vi "Calc Gain and Offset.vi"(9 "output cluster":T2, 10 "Count":u8, 11 "CalStatus":T1(ring)) -> (2 "New Count":u8, 3 "NewCalStatus":T1(ring))   [LabVIEW 2016]
uses:
  Controls/Cal Refs.ctl
  <vilib>/Analysis/baseanly.llb/Mean (DBL).vi
  <vilib>/Analysis/NI_AALBase.lvlib
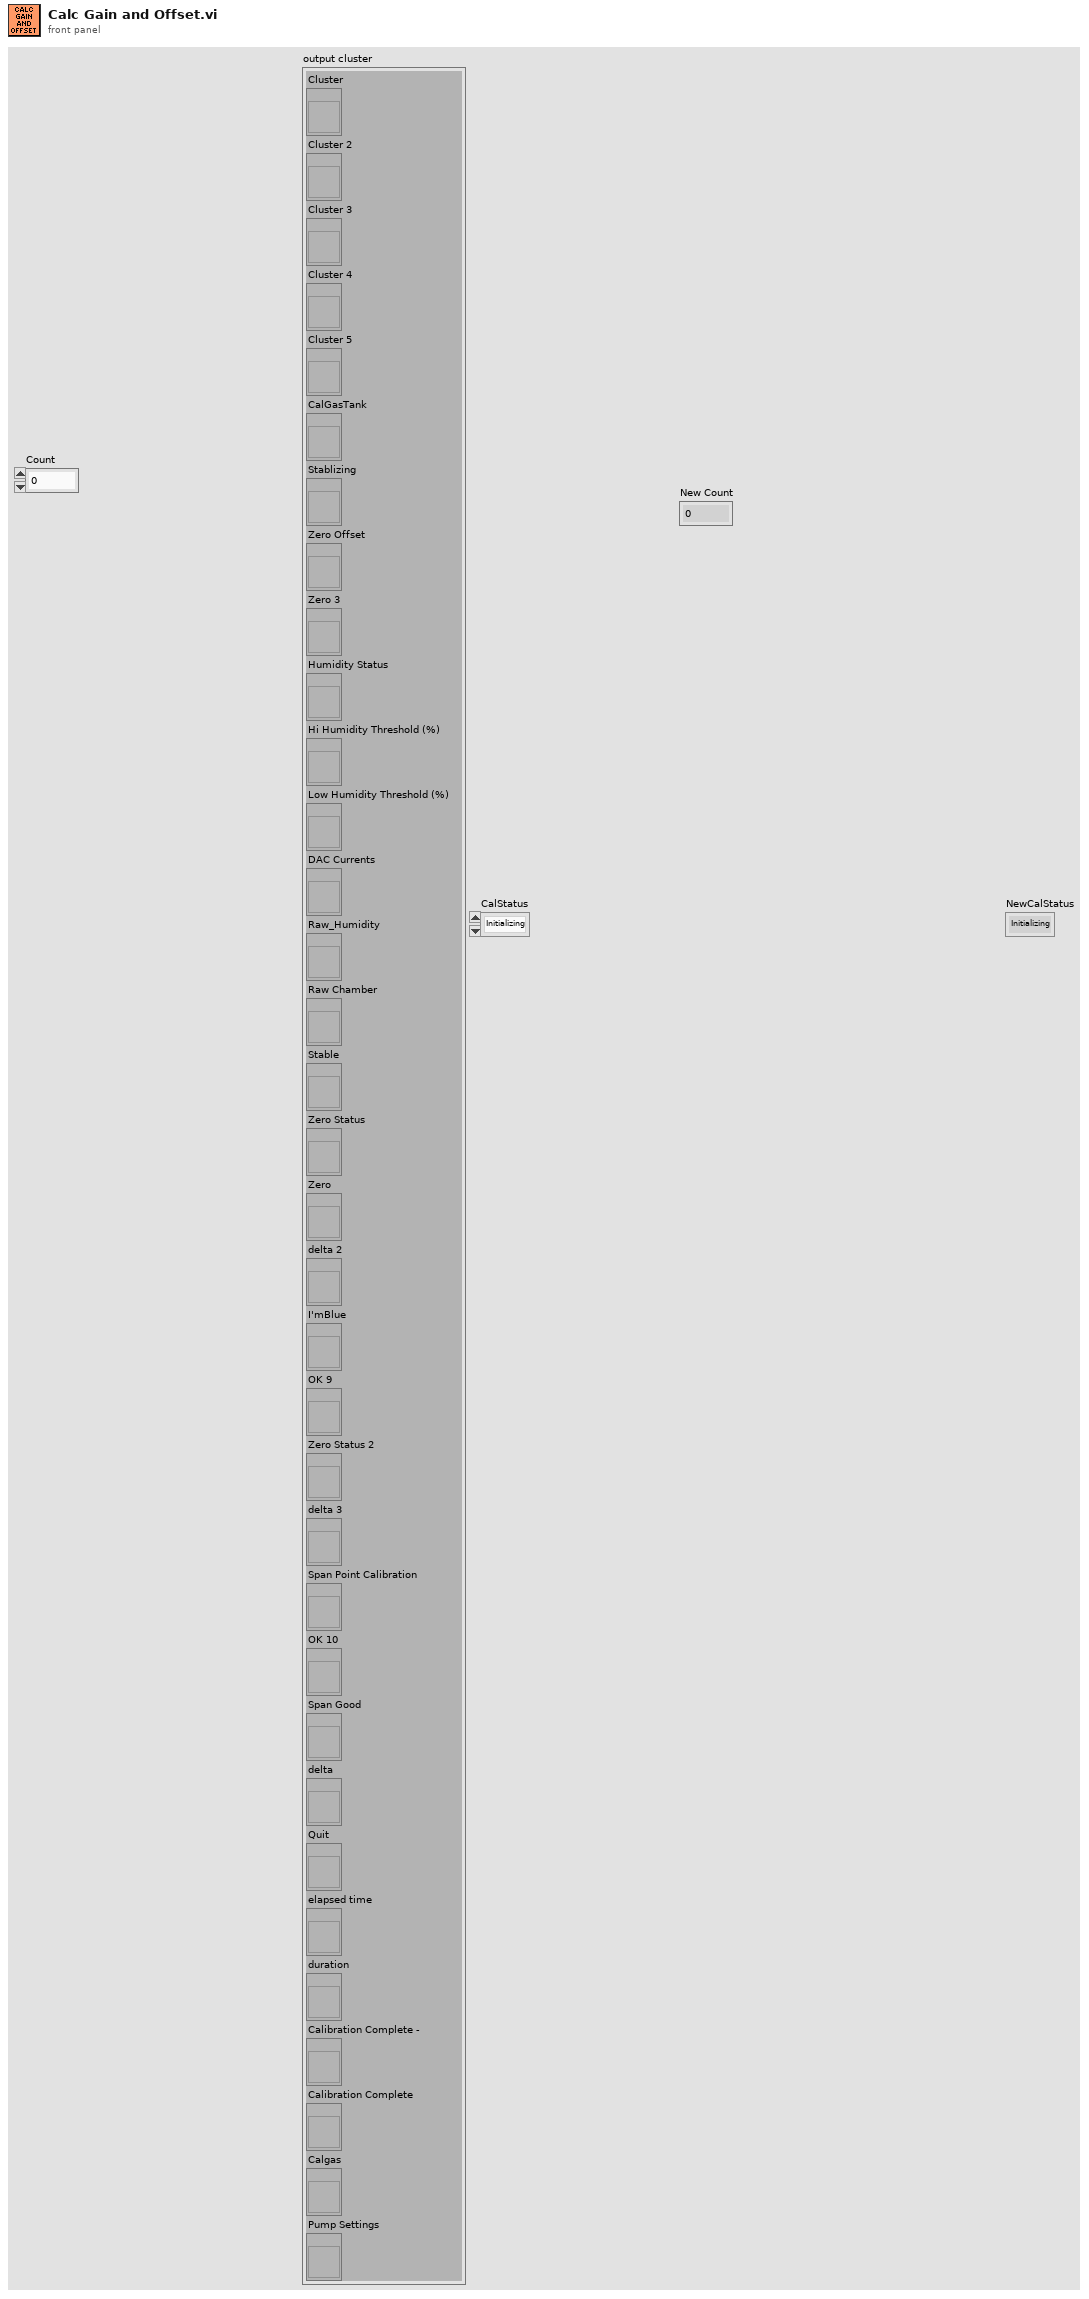
[diagram p1: front panel]
types:
  T1 = enum32{"Initializing", "Enter CO2 Value", "Enter Calibration Code", "Reading Calibration Data", "Stablizing", "Calculating Target Voltages", "Setting Zero Point", "Setting High Point", "Setting Span Point", "Calculating Gain & Offset", "Storing Calibration Coefficients", "Calibration Complete"}
  T2 = typedef "Cal Refs.ctl" = cluster{"Cluster":refnum<vi>, "Cluster 2":refnum<vi>, "Cluster 3":refnum<vi>, "Cluster 4":refnum<vi>, "Cluster 5":refnum<vi>, "CalGasTank":refnum<vi>, "Stablizing":refnum<vi>, "Zero Offset":refnum<vi>, "Zero 3":refnum<vi>, "Humidity Status":refnum<vi>, "Hi Humidity Threshold (%)":refnum<vi>, "Low Humidity Threshold (%)":refnum<vi>, "DAC Currents":refnum<vi>, "Raw_Humidity":refnum<vi>, "Raw Chamber":refnum<vi>, "Stable":refnum<vi>, "Zero Status":refnum<vi>, "Zero":refnum<vi>, "delta 2":refnum<vi>, "I'mBlue":refnum<vi>, "OK 9":refnum<vi>, "Zero Status 2":refnum<vi>, "delta 3":refnum<vi>, "Span Point Calibration":refnum<vi>, "OK 10":refnum<vi>, "Span Good":refnum<vi>, "delta":refnum<vi>, "Quit":refnum<vi>, "elapsed time":refnum<vi>, "duration":refnum<vi>, "Calibration Complete -":refnum<vi>, "Calibration Complete":refnum<vi>, "Calgas":refnum<vi>, "Pump Settings":refnum<vi>}
  T3 = cluster{"Tcal_Chamber":dbl, "Tcal_PCB":dbl, "Tcal_Film":dbl, "Tcal_Humidity":dbl, "Tcal_Det":dbl[], "Cal Gas":dbl, "Reference":dbl}
  T4 = cluster{"CalFile Selected":path, "TYPE":string, "DATE":string, "C0FC2V":dbl[], "C6FC2V":dbl[], "V_0d(target)":dbl[], "V_6d(target)":dbl[], "V_span(target)":dbl[], "CHANNEL":string[], "Status":bool[], "BlueLED 2":bool[], "C2V":u8[], "A":dbl[], "B":dbl[], "C":dbl[], "D":dbl[], "V2C":u8[], "A'":dbl[], "B'":dbl[], "C'":dbl[], "D'":dbl[]}
  T5 = cluster{"V_0d(ImA)\nActual":dbl[], "V_6d(ImA)\nActual":dbl[], "V_span(ImA)":dbl[], "V_0(adjust)\ncal offsets":dbl[], "V_span(adjust)":dbl[], "Gain(adjust)":dbl[]}
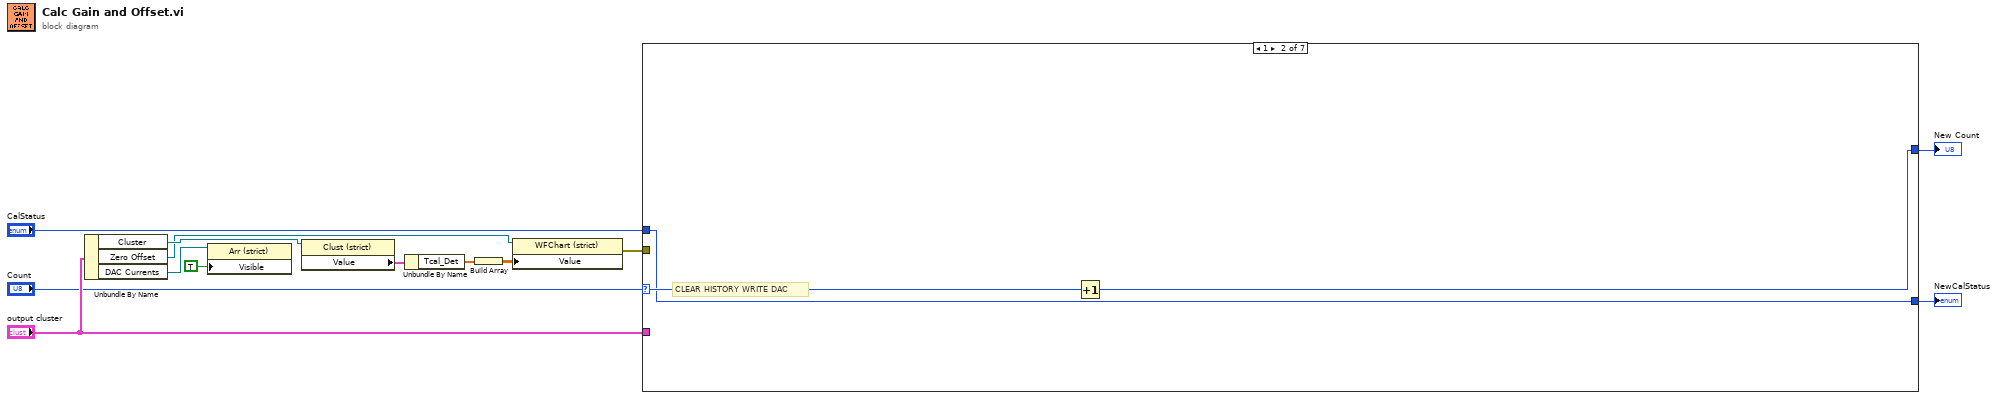
[diagram p0: block diagram]
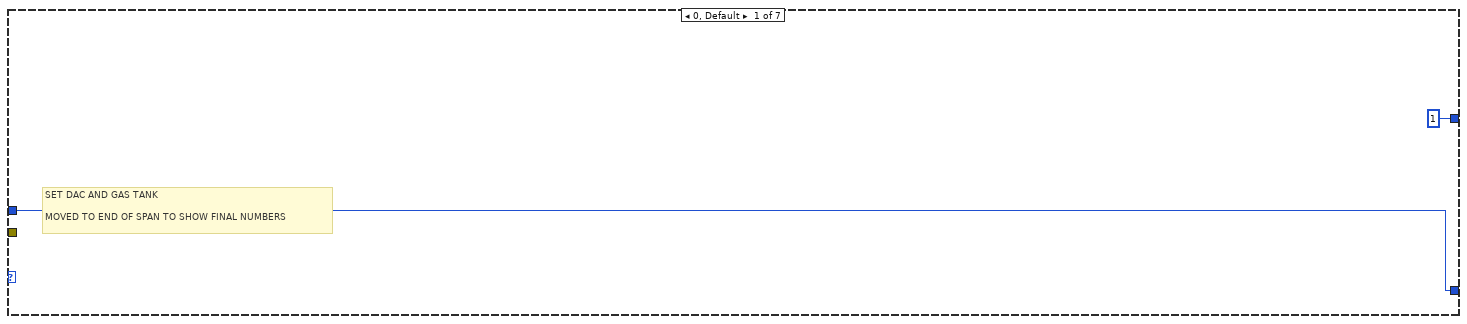
[diagram p2: hidden frame]
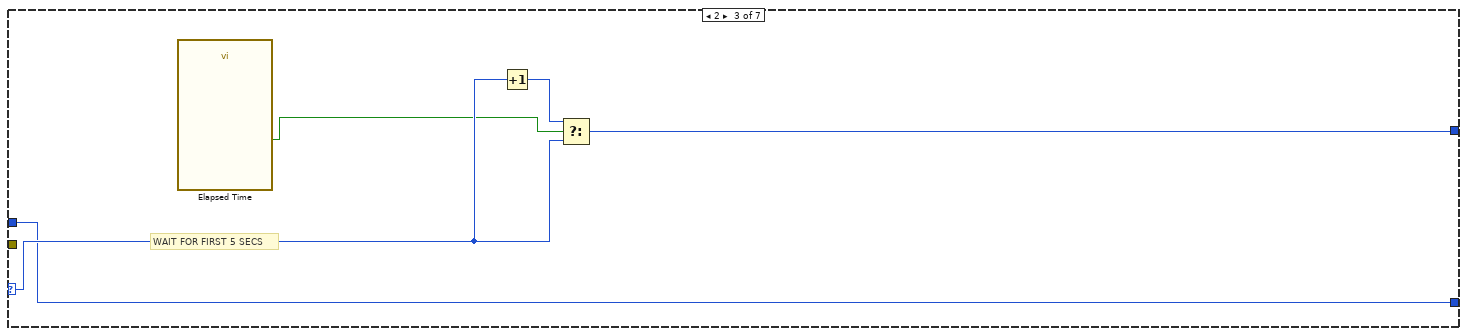
[diagram p3: hidden frame]
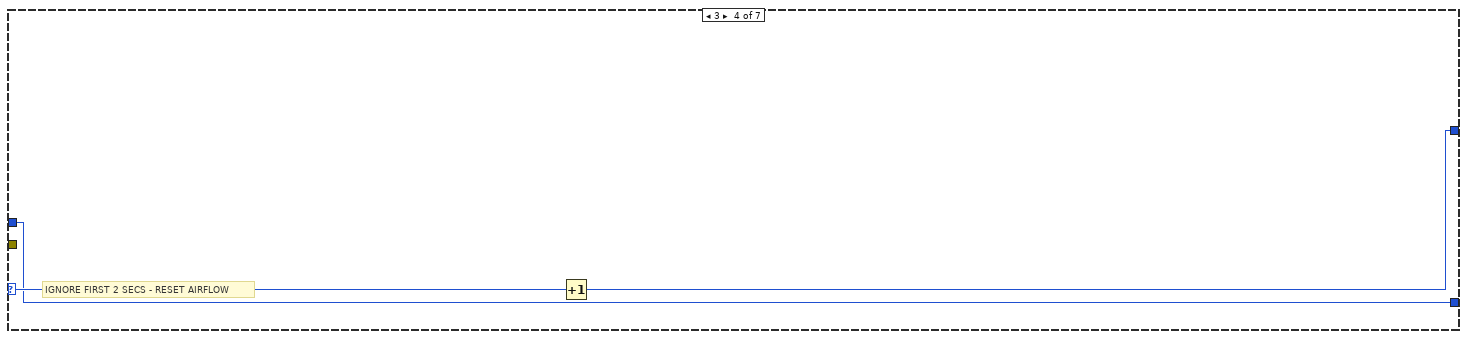
[diagram p4: hidden frame]
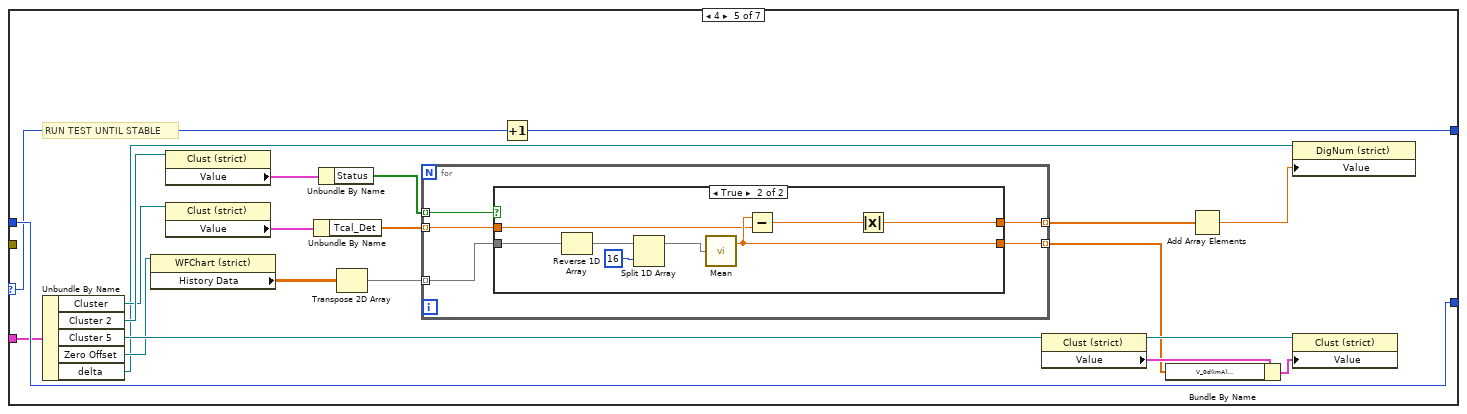
[diagram p5: hidden frame]
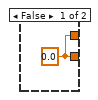
[diagram p6: hidden frame]
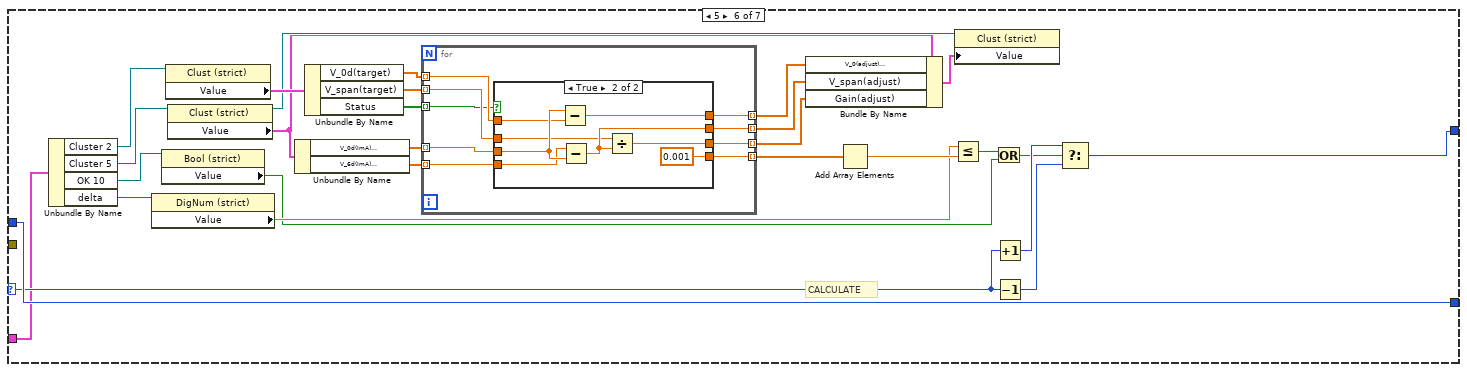
[diagram p7: hidden frame]
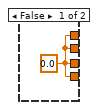
[diagram p8: hidden frame]
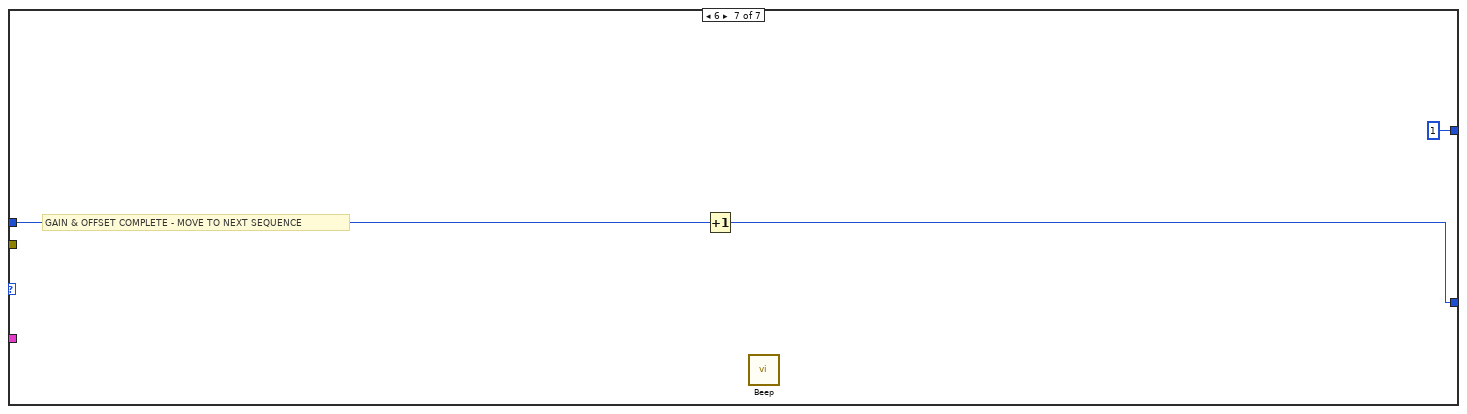
[diagram p9: hidden frame]
diagram:
  n1 = Unbundle By Name("output cluster") -> ("Cluster"=w8:refnum<vi>, "Zero Offset"=w7:refnum<vi>, "DAC Currents"=w9:refnum<vi>)
  n2 = property on="Property Node" class="Arr (strict)"(reference=w9, "Visible"=TRUE) -> ()  [unwired: 1 in, 2 out]
  n3 = property class="Clust (strict)"(reference=w8) -> ("Value"=w12:T3)  [unwired: 1 in, 2 out]
  n4 = Unbundle By Name(w12) -> ("Tcal_Det"=w11:dbl[])
  n5 = Build Array(w11) -> (w10:dbl[][])
  n6 = property class="WFChart (strict)"(reference=w7, "Value"=w10) -> (error out=w5:errorcluster)  [unwired: 1 in, 1 out]
  n7 = case shown="1" "Count" {
    selector: "Count" -> [_ w18 w23 w26 w46 w85 _]
    tunnel: [1 w17 w21 w24 w45 w88 1] -> w1
    tunnel: "CalStatus" -> [w15 w16 w20 w25 w47 w89 w110]
    tunnel: [w15 w16 w20 w25 w47 w89 w109] -> w3
    tunnel: "output cluster" -> [_ _ _ _ w37 w69 _]
    tunnel: w5 -> [_ _ _ _ _ _ _]
    frame 0, Default {
      # "SET DAC AND GAS TANK\n\nMOVED TO END OF SPAN TO SHOW FINAL NUMBERS"
    }
    frame 1 {
      # "CLEAR HISTORY WRITE DAC"
      n8 = Increment(x=w18) -> (x+1=w17:u8)
    }
    frame 2 {
      # "WAIT FOR FIRST 5 SECS"
      n9 = call "Elapsed Time"() -> ("Time has Elapsed"=w19:bool)  [unwired: 12 in, 7 out]
      n10 = Increment(x=w23) -> (x+1=w22:u8)
      n11 = Select(t=w22, s=w19, f=w23) -> (s? t:f=w21:u8)
    }
    frame 3 {
      # "IGNORE FIRST 2 SECS - RESET AIRFLOW"
      n12 = Increment(x=w26) -> (x+1=w24:u8)
    }
    frame 4 {
      # "RUN TEST UNTIL STABLE"
      n13 = Unbundle By Name(w37) -> ("Cluster"=w31:refnum<vi>, "Cluster 2"=w34:refnum<vi>, "Cluster 5"=w36:refnum<vi>, "Zero Offset"=w28:refnum<vi>, "delta"=w27:refnum<vi>)
      n14 = property on="Property Node" class="WFChart (strict)"(reference=w28) -> ("History Data"=w44:dbl[][])  [unwired: 1 in, 2 out]
      n15 = property class="Clust (strict)"(reference=w34) -> ("Value"=w35:T4)  [unwired: 1 in, 2 out]
      n16 = property class="Clust (strict)"(reference=w31) -> ("Value"=w32:T3)  [unwired: 1 in, 2 out]
      n17 = Unbundle By Name(w32) -> ("Tcal_Det"=w30:dbl[])
      n18 = Unbundle By Name(w35) -> ("Status"=w33:bool[])
      n19 = Transpose 2D Array(2D array=w44) -> (transposed array=w43:dbl[][])
      n20 = for {
        tunnel: w43 -> [w52] mode=indexing
        tunnel: [w51] -> w38 mode=indexing
        tunnel: w30 -> [w50] mode=indexing
        tunnel: [w49] -> w42 mode=indexing
        tunnel: w33 -> [w48] mode=indexing
        n21 = case shown="True" w48 {
          tunnel: w52 -> [_ w57]
          tunnel: [w53 w56] -> w51
          tunnel: w50 -> [_ w55]
          tunnel: [w53 w54] -> w49
          frame False {
            w53 = 0.0 ("mean")
          }
          frame True {
            n22 = Reverse 1D Array(array=w57) -> (reversed array=w58:dbl[])
            n23 = Split 1D Array(array=w58, index=16) -> (first subarray=w59:dbl[])  [unwired: 1 out]
            n24 = call-poly <vilib>:"Mean.vi"("X"=w59) -> ("mean"=w56:dbl)  [unwired: 1 out]
            n25 = Subtract(x=w56, y=w55) -> (x-y=w61:dbl)
            n26 = Absolute Value(x=w61) -> (abs(x)=w54:dbl)
          }
        }
      }
      n27 = Increment(x=w46) -> (x+1=w45:u8)
      n28 = property class="Clust (strict)"(reference=w36) -> (reference out=w41:refnum<vi>, "Value"=w40:T5)  [unwired: 1 in, 1 out]
      n29 = Bundle By Name(cluster=w40, "V_0d(ImA)\nActual"=w38) -> (w39:T5)
      n30 = Add Array Elements(numeric array=w42) -> (sum=w29:dbl)
      n31 = property class="DigNum (strict)"(reference=w27, "Value"=w29) -> ()  [unwired: 1 in, 2 out]
      n32 = property class="Clust (strict)"(reference=w41, "Value"=w39) -> ()  [unwired: 1 in, 2 out]
    }
    frame 5 {
      # "CALCULATE"
      n33 = Unbundle By Name(w69) -> ("Cluster 2"=w67:refnum<vi>, "Cluster 5"=w68:refnum<vi>, "OK 10"=w64:refnum<vi>, "delta"=w62:refnum<vi>)
      n34 = property class="DigNum (strict)"(reference=w62) -> ("Value"=w65:dbl)  [unwired: 1 in, 2 out]
      n35 = property class="Bool (strict)"(reference=w64) -> ("Value"=w63:bool)  [unwired: 1 in, 2 out]
      n36 = property class="Clust (strict)"(reference=w67) -> ("Value"=w80:T4)  [unwired: 1 in, 2 out]
      n37 = property class="Clust (strict)"(reference=w68) -> (reference out=w74:refnum<vi>, "Value"=w73:T5)  [unwired: 1 in, 1 out]
      n38 = Unbundle By Name(w73) -> ("V_0d(ImA)\nActual"=w77:dbl[], "V_6d(ImA)\nActual"=w76:dbl[])
      n39 = Unbundle By Name(w80) -> ("V_0d(target)"=w79:dbl[], "V_span(target)"=w78:dbl[], "Status"=w66:bool[])
      n40 = for {
        tunnel: [w98] -> w70 mode=indexing
        tunnel: [w97] -> w71 mode=indexing
        tunnel: [w96] -> w72 mode=indexing
        tunnel: w77 -> [w95] mode=indexing
        tunnel: w78 -> [w94] mode=indexing
        tunnel: w79 -> [w93] mode=indexing
        tunnel: w76 -> [w92] mode=indexing
        tunnel: [w91] -> w82 mode=indexing
        tunnel: w66 -> [w90] mode=indexing
        n41 = case shown="True" w90 {
          tunnel: [w99 w107] -> w98
          tunnel: [w99 w106] -> w97
          tunnel: [w99 w105] -> w96
          tunnel: w95 -> [_ w104]
          tunnel: w94 -> [_ w103]
          tunnel: w93 -> [_ w102]
          tunnel: w92 -> [_ w101]
          tunnel: [w99 0.001] -> w91
          frame False {
            w99 = 0.0
          }
          frame True {
            n42 = Subtract(x=w104, y=w102) -> (x-y=w105:dbl)
            n43 = Subtract(x=w101, y=w104) -> (x-y=w106:dbl)
            n44 = Divide(x=w103, y=w106) -> (x/y=w107:dbl)
          }
        }
      }
      n45 = Bundle By Name(cluster=w73, "V_0(adjust)\ncal offsets"=w72, "V_span(adjust)"=w71, "Gain(adjust)"=w70) -> (w75:T5)
      n46 = Add Array Elements(numeric array=w82) -> (sum=w81:dbl)
      n47 = Less Or Equal?(x=w65, y=w81) -> (x <= y?=w84:bool)
      n48 = property class="Clust (strict)"(reference=w74, "Value"=w75) -> ()  [unwired: 1 in, 2 out]
      n49 = Or(x=w84, y=w63) -> (x .or. y?=w83:bool)
      n50 = Increment(x=w85) -> (x+1=w87:u8)
      n51 = Decrement(x=w85) -> (x-1=w86:u8)
      n52 = Select(t=w87, s=w83, f=w86) -> (s? t:f=w88:u8)
    }
    frame 6 {
      # "GAIN & OFFSET COMPLETE - MOVE TO NEXT SEQUENCE"
      n53 = Increment(x=w110) -> (x+1=w109:T1)
      n54 = call <vilib>:"Beep.vi"() -> ()  [unwired: 12 in]
    }
  }
  "NewCalStatus" <- w3
  "New Count" <- w1
